vi "Get Device Information.vi"(8 "error in (no error)":errorcluster, 11 "Potentiostat Galvanostat in":refnum<class "Potentiostat Galvanostat.lvclass">) -> (0 "error out":errorcluster, 1 "Device Information":T1 {"Device Code" items=["VMP device"=0, "VMP2 device"=1, "MPG device"=2, "BISTAT device"=3, "MCS-200 device"=4, "VMP3 device"=5, "VSP"=6, "HCP-803"=7, "EPP-400"=8, "EPP-4000"=9, "BISTAT 2"=10, "FCT-150S"=11, "VMP-300"=12, "SP-50"=13, "SP-150"=14, "FCT-50S"=15, "SP300"=16, "CLB-500"=17, "HCP-1005"=18, "CLB-2000"=19, "VSP-300"=20, "SP-200"=21, "MPG2"=22, "SP-100"=23, "MOSLED"=24, "Kinetic device... \\warning unused code"=25, "Nikita"=26, "SP-240"=27, "MPG-205 (techno VMP3) \\warning not controled by kernel2"=28, "MPG-210 (techno VMP3) \\warning not controled by kernel2"=29, "MPG-220 (techno VMP3) \\warning not controled by kernel2"=30, "MPG-240 (techno VMP3) \\warning not controled by kernel2"=31, "BP-300"=32, "VMP-3e  (VMP3)"=33, "VSP-3e  (VMP3)"=34, "SP-50e  (VMP3)"=35, "SP-150e (VMP3)"=36, "Unknown device"=255]}, 3 "Potentiostat Galvanostat out":refnum<class "Potentiostat Galvanostat.lvclass">)   [LabVIEW 2018, in "Potentiostat Galvanostat.lvclass"]
uses:
  Potentiostat Galvanostat.lvclass
  Potentiostat Galvanostat.lvclass/Potentiostat Galvanostat.ctl
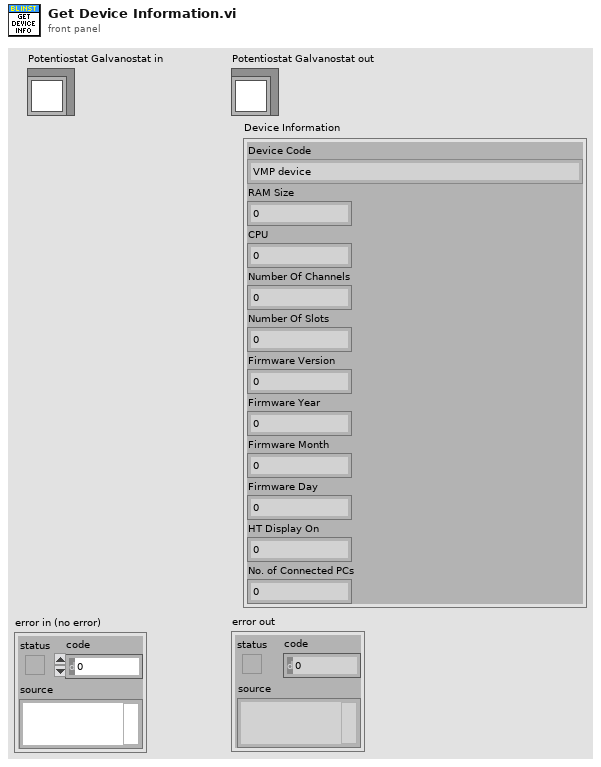
[diagram p1: front panel]
types:
  T1 = cluster{"Device Code":i32, "RAM Size":i32, "CPU":i32, "Number Of Channels":i32, "Number Of Slots":i32, "Firmware Version":i32, "Firmware Year":i32, "Firmware Month":i32, "Firmware Day":i32, "HT Display On":i32, "No. of Connected PCs":i32}
  T2 = typedef "Potentiostat Galvanostat.lvclass/Device Information.ctl" = cluster{"Device Code":T3, "RAM Size":i32, "CPU":i32, "Number Of Channels":i32, "Number Of Slots":i32, "Firmware Version":i32, "Firmware Year":i32, "Firmware Month":i32, "Firmware Day":i32, "HT Display On":i32, "No. of Connected PCs":i32}
  T3 = typedef "Potentiostat Galvanostat.lvclass/Device Code.ctl" = i32
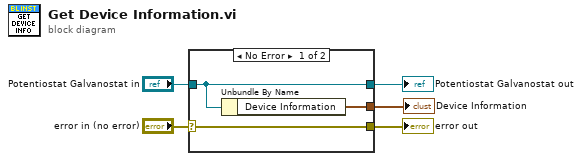
[diagram p0: block diagram]
diagram:
  n1 = case shown="No Error" "error in (no error)" {
    selector: "error in (no error)" -> [w8 w9]
    tunnel: [w8 w9] -> w4
    tunnel: [w7 w10] -> w2
    tunnel: "Potentiostat Galvanostat in" -> [w7 w10]
    tunnel: [w6 _] -> w1
    frame No Error {
      n2 = Unbundle By Name(w7) -> ("Device Information"=w6:T2)
    }
    frame Error {
    }
  }
  "error out" <- w4
  "Potentiostat Galvanostat out" <- w2
  "Device Information" <- w1
